vi "K2450 Set Current.vi"(8 "error in (no error)":errorcluster {"code" format="%.0x"}, 10 "Current 2450":dbl, 11 "VISA resource name":refnum<visa-resource-name>) -> (0 "error out":errorcluster {"code" format="%.0x"}, 3 "dup VISA Session":refnum<visa-resource-name>)   [LabVIEW 2025]
doc: "Author: Scott Hannahs <sth@magnet.fsu.edu>\n\nThis software is licensed for use under the “MIT License\"\nCopyright (c) 2025 Scott Hannahs, sth@sth@magnet.sthnet.net\n\nPermission is hereby granted, free of charge, to any person obtaining a copy of this software and associated documentation files (the \"Software\"), to deal in the Software without restriction, including without limitation the rights to use, copy, modify, merge, publish, distribute, sublicense, and/or sell copies of the Software, and to permit persons to whom the Software is furnished to do so, subject to the following conditions: The above copyright notice and this permission notice shall be included in all copies or substantial portions of the Software.\n\nTHE SOFTWARE IS PROVIDED \"AS IS\", WITHOUT WARRANTY OF ANY KIND, EXPRESS OR IMPLIED, INCLUDING BUT NOT LIMITED TO THE WARRANTIES OF MERCHANTABILITY, FITNESS FOR A PARTICULAR PURPOSE AND NONINFRINGEMENT. IN NO EVENT SHALL THE AUTHORS OR COPYRIGHT HOLDERS BE LIABLE FOR ANY CLAIM, DAMAGES OR OTHER LIABILITY, WHETHER IN AN ACTION OF CONTRACT, TORT OR OTHERWISE, ARISING FROM, OUT OF OR IN CONNECTION WITH THE SOFTWARE OR THE USE OR OTHER DEALINGS IN THE SOFTWARE."
panel:
  # "Make sure unit is set to source Current\nsour:func Curr\nAnd turned on\nOUTPut ON"
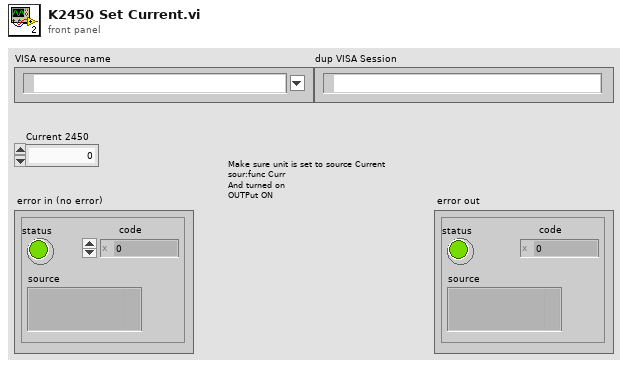
[diagram p1: front panel]
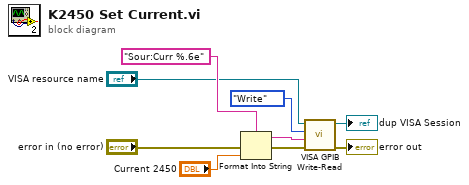
[diagram p0: block diagram]
diagram:
  n1 = Format Into String(format string="Sour:Curr %.6e" ("Command"), error in="error in (no error)", "Current 2450") -> (resulting string=w5:string, error out=w3:errorcluster)  [unwired: 1 in]
  n2 = call "VISA GPIB Write-Read.vi"("error in (no error)"=w3, "Command"=w5, "Action"=enum16{"Write", "Read", "Write & Read"}."Write", "VISA resource name"="VISA resource name") -> ("error out"=→"error out":errorcluster, "dup VISA Session"=→"dup VISA Session":refnum<visa-resource-name>)  [unwired: 4 in, 2 out]
